vi "crdCalcExtinction.vi"(9 "R_l":dbl, 10 "tau_0 (us)":dbl, 11 "tau (us)":dbl) -> (3 "b_ext (1/Mm)":dbl)   [LabVIEW 2011]
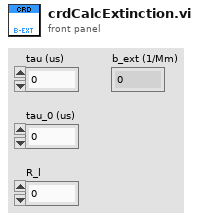
[diagram p1: front panel]
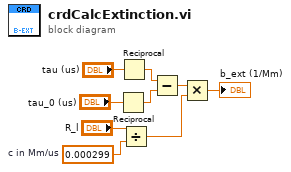
[diagram p0: block diagram]
diagram:
  w4 = 0.000299  # c in Mm/us
  n1 = Reciprocal(x="tau_0 (us)") -> (1/x=w6:dbl)
  n2 = Reciprocal(x="tau (us)") -> (1/x=w5:dbl)
  n3 = Divide(x="R_l", y=w4) -> (x/y=w8:dbl)
  n4 = Subtract(x=w5, y=w6) -> (x-y=w7:dbl)
  n5 = Multiply(x=w7, y=w8) -> (x*y=→"b_ext (1/Mm)":dbl)
